vi "py.create.Pitch.vi"(8 "error in (no error)":errorcluster, 11 "Parameters":variant) -> (0 "error out":errorcluster, 3 "bytes":u8[](array[numeric]) format="%.0x")   [LabVIEW 2020]
uses:
  AddOrder/AddOrderLong.Parameters.ctl
  Time/Time.Parameters.ctl
  OrderExecuted/OrderExecuted.Parameters.ctl
  ReduceSize/ReduceSizeLong.Parameters.ctl
  ReduceSize/ReduceSizeShort.Parameters.ctl
  ModifyOrder/ModifyOrderLong.Parameters.ctl
  ModifyOrder/ModifyOrderShort.Parameters.ctl
  DeleteOrder/DeleteOrder.Parameters.ctl
  Trade/TradeLong.Parameters.ctl
  Trade/TradeShort.Parameters.ctl
  Trade/TradeExpanded.Parameters.ctl
  AddOrder/AddOrderShort.Parameters.ctl
  AddOrder/AddOrderExpanded.Parameters.ctl
  OrderExecuted/OrderExecutedAtPriceSize.Parameters.ctl
  <vilib>/Utility/Data Type/NI_Data Type.lvlib
  AddOrder/AddOrderLong.lvclass
  Time/Time.lvclass
  OrderExecuted/OrderExecuted.lvclass
  ReduceSize/ReduceSizeLong.lvclass
  ReduceSize/ReduceSizeShort.lvclass
  ModifyOrder/ModifyOrderLong.lvclass
  ModifyOrder/ModifyOrderShort.lvclass
  DeleteOrder/DeleteOrder.lvclass
  Trade/TradeLong.lvclass
  Trade/TradeShort.lvclass
  Trade/TradeExpanded.lvclass
  AddOrder/AddOrderShort.lvclass
  AddOrder/AddOrderExpanded.lvclass
  OrderExecuted/OrderExecutedAtPriceSize.lvclass
panel:
  out "Application Directory":path
  out "name":string
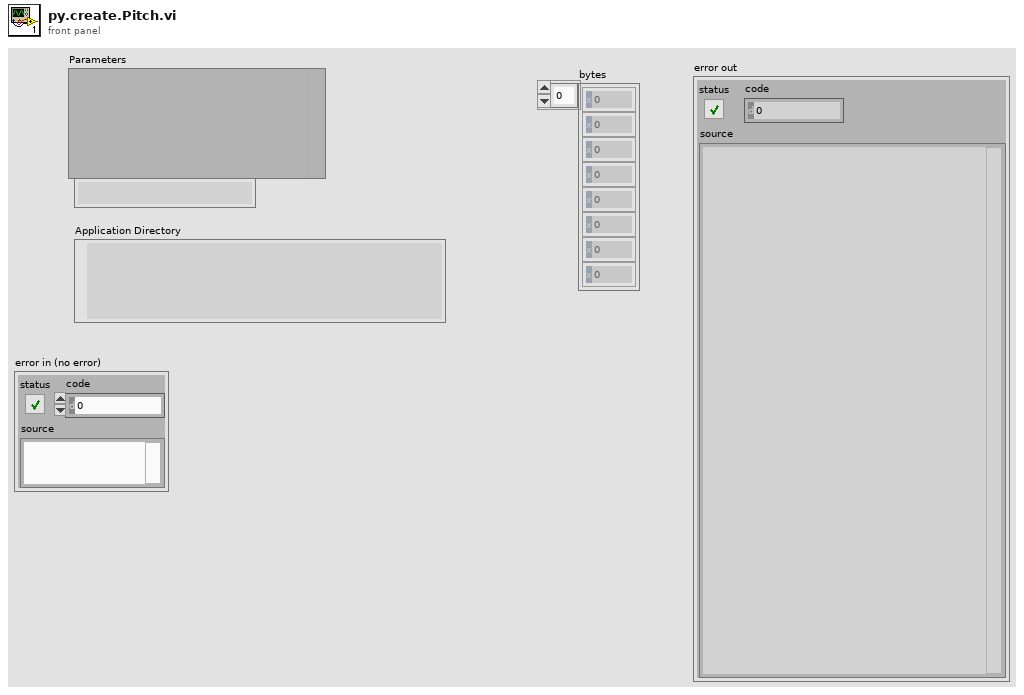
[diagram p1: front panel]
types:
  T1 = typedef "AddOrderLong.lvclass/AddOrderLong.Parameters.ctl" = cluster{"Time Offset":u32, "Order Id":string, "Quantity":u32, "Symbol":string, "Side Indicator":string, "Price":dbl}
  T2 = typedef "Time.lvclass/Time.Parameters.ctl" = cluster{"Time":u32}
  T3 = typedef "OrderExecuted.lvclass/OrderExecuted.Parameters.ctl" = cluster{"Time Offset":u32, "Order Id":string, "Executed Quantity":u32, "Execution Id":string}
  T4 = typedef "ReduceSizeLong.lvclass/ReduceSizeLong.Parameters.ctl" = cluster{"Time Offset":u32, "Order Id":string, "Canceled Quantity":u32}
  T5 = typedef "ReduceSizeShort.lvclass/ReduceSizeShort.Parameters.ctl" = cluster{"Time Offset":u32, "Order Id":string, "Canceled Quantity":u16}
  T6 = typedef "ModifyOrderLong.lvclass/ModifyOrderLong.Parameters.ctl" = cluster{"Time Offset":u32, "Order Id":string, "Quantity":u32, "Price":dbl, "Modify Flags":u8}
  T7 = typedef "ModifyOrderShort.lvclass/ModifyOrderShort.Parameters.ctl" = cluster{"Time Offset":u32, "Order Id":string, "Quantity":u32, "Price":u16, "Modify Flags":u8}
  T8 = typedef "DeleteOrder.lvclass/DeleteOrder.Parameters.ctl" = cluster{"Time Offset":u32, "Order Id":string}
  T9 = typedef "TradeLong.lvclass/TradeLong.Parameters.ctl" = cluster{"Time Offset":u32, "Order Id":string, "Execution Id":string, "Quantity":u32, "Price":dbl, "Side Indicator":string, "Symbol":string}
  T10 = typedef "TradeShort.lvclass/TradeShort.Parameters.ctl" = cluster{"Time Offset":u32, "Order Id":string, "Execution Id":string, "Quantity":u32, "Price":dbl, "Side Indicator":string, "Symbol":string}
  T11 = typedef "TradeExpanded.lvclass/TradeExpanded.Parameters.ctl" = cluster{"Time Offset":u32, "Order Id":string, "Side Indicator":string, "Quantity":u32, "Symbol":string, "Price":dbl, "Execution Id":string}
  T12 = typedef "AddOrderShort.lvclass/AddOrderShort.Parameters.ctl" = cluster{"Time Offset":u32, "Order Id":string, "Quantity":u32, "Symbol":string, "Side Indicator":string, "Price":dbl}
  T13 = typedef "AddOrderExpanded.lvclass/AddOrderExpanded.Parameters.ctl" = cluster{"Time Offset":u32, "Order Id":string, "Quantity":u32, "Symbol":string, "Side Indicator":string, "Price":dbl, "Participant Id":string, "Customer Indicator":string}
  T14 = typedef "OrderExecutedAtPriceSize.lvclass/OrderExecutedAtPriceSize.Parameters.ctl" = cluster{"Time Offset":u32, "Order Id":string, "Executed Quantity":u32, "Execution Id":string, "Remaining Quantity":u32, "Price":dbl}
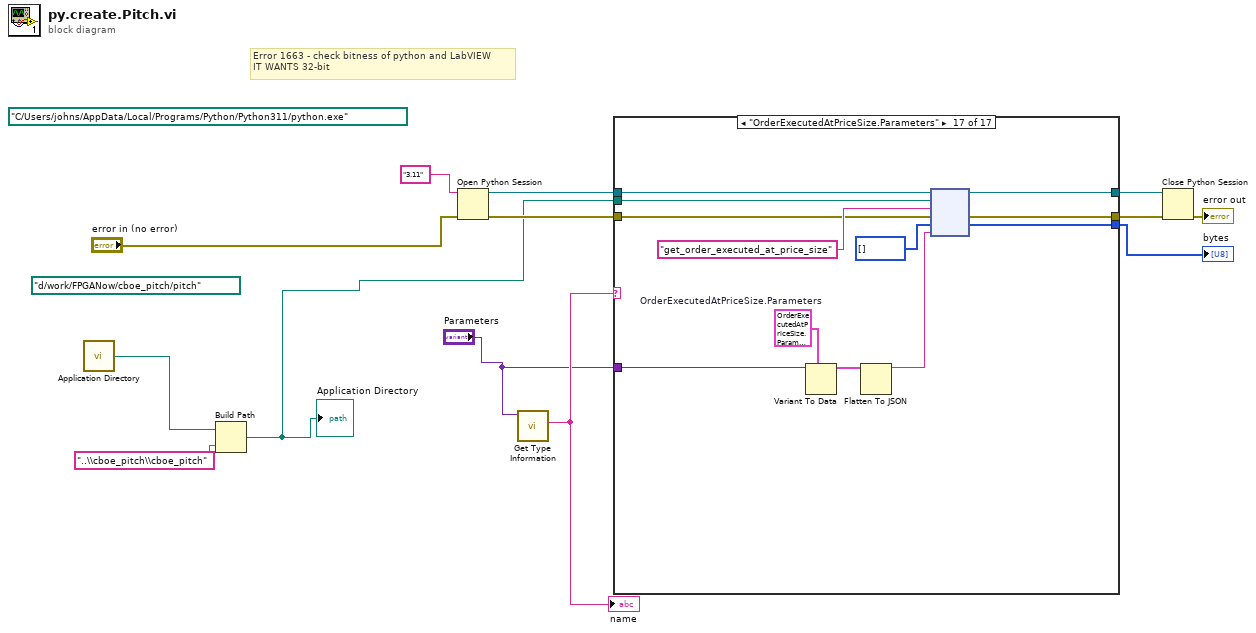
[diagram p0: block diagram]
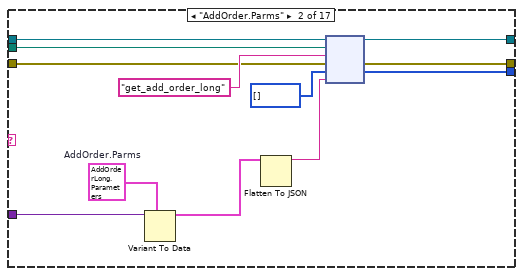
[diagram p3: hidden frame]
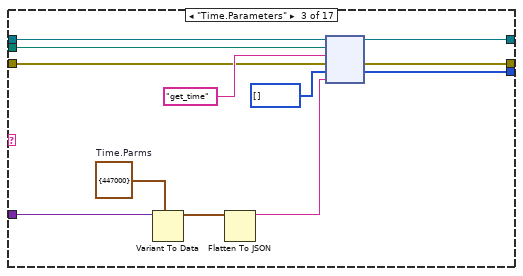
[diagram p4: hidden frame]
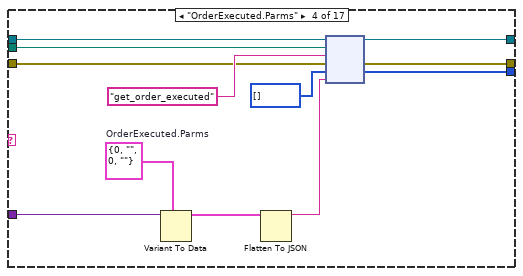
[diagram p5: hidden frame]
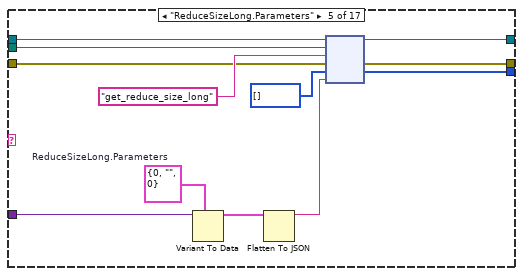
[diagram p6: hidden frame]
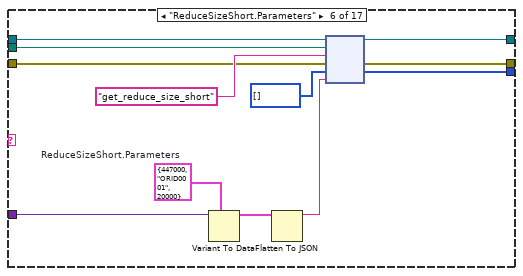
[diagram p7: hidden frame]
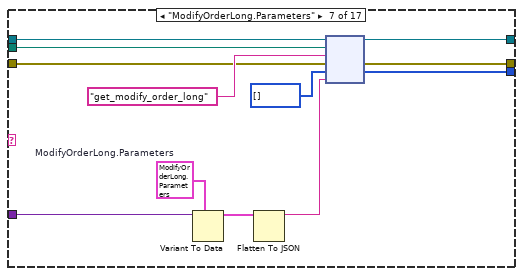
[diagram p8: hidden frame]
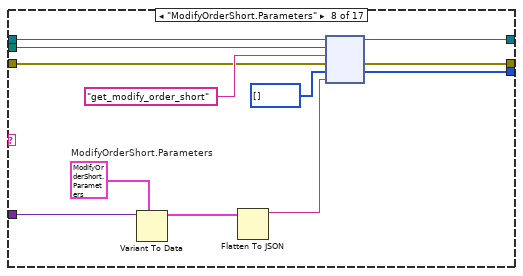
[diagram p9: hidden frame]
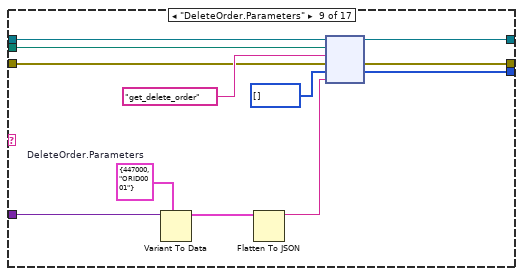
[diagram p10: hidden frame]
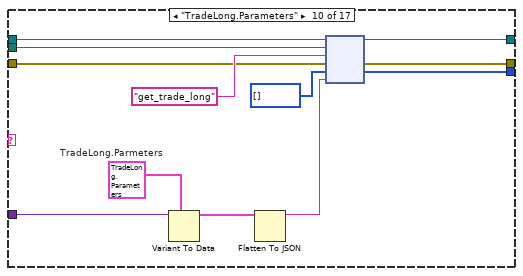
[diagram p11: hidden frame]
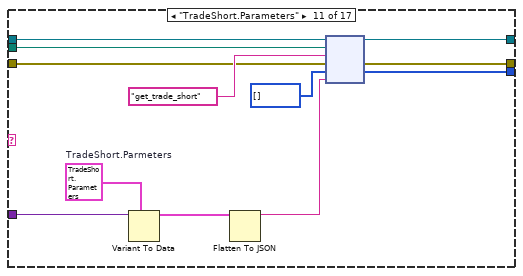
[diagram p12: hidden frame]
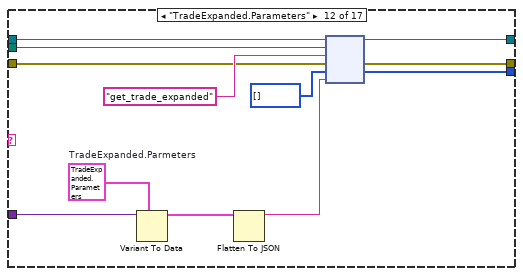
[diagram p13: hidden frame]
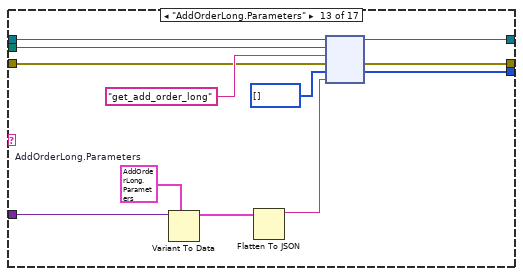
[diagram p14: hidden frame]
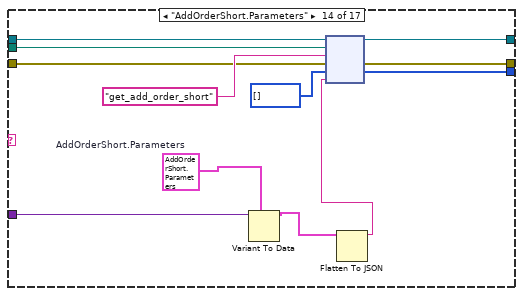
[diagram p15: hidden frame]
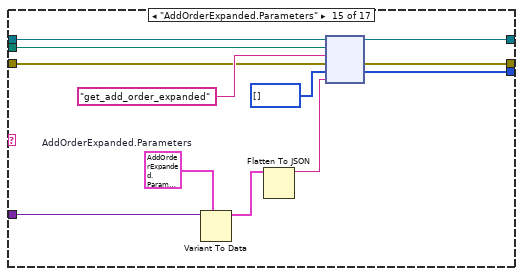
[diagram p16: hidden frame]
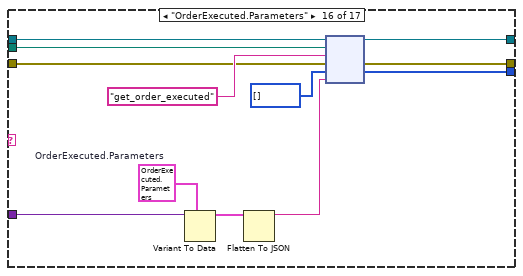
[diagram p17: hidden frame]
diagram:
  (unwired) path "C:/Users/johns/AppData/Local/Programs/Python/Python311/python.exe" ("Python path")
  (unwired) path "d:/work/FPGANow/cboe_pitch/pitch" ("module path")
  # "Error 1663 - check bitness of python and LabVIEW\nIT WANTS 32-bit"
  n1 = call <vilib>:"Application Directory.vi"() -> ("Application Directory"=w6:path)
  n2 = Build Path(base path=w6, name or relative path="..\\cboe_pitch\\cboe_pitch") -> (appended path=w4:path)
  "Application Directory" <- w4
  n3 = Open Python Session(python version="3.11" ("Python version"), 3:"error in (no error)") -> (session out=w3:refnum<k35>, error out=w10:errorcluster)  [unwired: 1 in]
  n4 = call <vilib>:"Get Type Information.vi"("variant"="Parameters") -> ("name"=w2:string)  [unwired: 6 in, 4 out]
  "name" <- w2
  n5 = case shown="\"OrderExecutedAtPriceSize.Parameters\"" w2 {
    tunnel: w3 -> [w15 w27 w39 w51 w63 w75 w87 w99 w111 w123 w135 w147 w159 w171 w183 w195 w207]
    tunnel: [w15 w26 w38 w50 w62 w74 w86 w98 w110 w122 w134 w146 w158 w170 w182 w194 w206] -> w13
    tunnel: w4 -> [_ w25 w37 w49 w61 w73 w85 w97 w109 w121 w133 w145 w157 w169 w181 w193 w205]
    tunnel: [w14 w24 w36 w48 w60 w72 w84 w96 w108 w120 w132 w144 w156 w168 w180 w192 w204] -> w11
    tunnel: w10 -> [w14 w22 w34 w46 w58 w70 w82 w94 w106 w118 w130 w142 w154 w166 w178 w190 w202]
    tunnel: [_ w21 w33 w45 w57 w69 w81 w93 w105 w117 w129 w141 w153 w165 w177 w189 w201] -> w9
    tunnel: "Parameters" -> [_ w19 w31 w43 w55 w67 w79 w91 w103 w115 w127 w139 w151 w163 w174 w187 w199]
    frame "False", Default {
    }
    frame "AddOrder.Parms" {
      w18 = T1 {"Time Offset"=447000, "Order Id"="ORID0001", "Quantity"=20000, "Symbol"="AAPL", "Side Indicator"="B", "Price"=0.905}  # AddOrder.Parms
      n6 = Variant To Data(type=w18, Variant=w19) -> (data=w17:T1)  [unwired: 1 in, 1 out]
      n7 = Flatten To JSON(anything=w17) -> (JSON string=w16:string)  [unwired: 2 in, 1 out]
      n8 = node(w27, w25, "get_add_order_long" ("function name"), w22, u8[] [], w16) -> (w26:refnum<k35>, w24:errorcluster, w21:u8[])  [unwired: 1 in, 2 out]
    }
    frame "Time.Parameters" {
      w30 = T2 {"Time"=447000}  # Time.Parms
      n9 = Variant To Data(type=w30, Variant=w31) -> (data=w29:T2)  [unwired: 1 in, 1 out]
      n10 = Flatten To JSON(anything=w29) -> (JSON string=w28:string)  [unwired: 2 in, 1 out]
      n11 = node(w39, w37, "get_time" ("function name"), w34, u8[] [], w28) -> (w38:refnum<k35>, w36:errorcluster, w33:u8[])  [unwired: 1 in, 2 out]
    }
    frame "OrderExecuted.Parms" {
      w42 = T3 {"Time Offset"=0, "Order Id"="", "Executed Quantity"=0, "Execution Id"=""}  # OrderExecuted.Parms
      n12 = Variant To Data(type=w42, Variant=w43) -> (data=w41:T3)  [unwired: 1 in, 1 out]
      n13 = Flatten To JSON(anything=w41) -> (JSON string=w40:string)  [unwired: 2 in, 1 out]
      n14 = node(w51, w49, "get_order_executed" ("function name"), w46, u8[] [], w40) -> (w50:refnum<k35>, w48:errorcluster, w45:u8[])  [unwired: 1 in, 2 out]
    }
    frame "ReduceSizeLong.Parameters" {
      w54 = T4 {"Time Offset"=0, "Order Id"="", "Canceled Quantity"=0}  # ReduceSizeLong.Parameters
      n15 = Variant To Data(type=w54, Variant=w55) -> (data=w53:T4)  [unwired: 1 in, 1 out]
      n16 = Flatten To JSON(anything=w53) -> (JSON string=w52:string)  [unwired: 2 in, 1 out]
      n17 = node(w63, w61, "get_reduce_size_long" ("function name"), w58, u8[] [], w52) -> (w62:refnum<k35>, w60:errorcluster, w57:u8[])  [unwired: 1 in, 2 out]
    }
    frame "ReduceSizeShort.Parameters" {
      w66 = T5 {"Time Offset"=447000, "Order Id"="ORID0001", "Canceled Quantity"=20000}  # ReduceSizeShort.Parameters
      n18 = Variant To Data(type=w66, Variant=w67) -> (data=w65:T5)  [unwired: 1 in, 1 out]
      n19 = Flatten To JSON(anything=w65) -> (JSON string=w64:string)  [unwired: 2 in, 1 out]
      n20 = node(w75, w73, "get_reduce_size_short" ("function name"), w70, u8[] [], w64) -> (w74:refnum<k35>, w72:errorcluster, w69:u8[])  [unwired: 1 in, 2 out]
    }
    frame "ModifyOrderLong.Parameters" {
      w78 = T6 {"Time Offset"=447000, "Order Id"="ORID0001", "Quantity"=20000, "Price"=0.905, "Modify Flags"=1}  # ModifyOrderLong.Parameters
      n21 = Variant To Data(type=w78, Variant=w79) -> (data=w77:T6)  [unwired: 1 in, 1 out]
      n22 = Flatten To JSON(anything=w77) -> (JSON string=w76:string)  [unwired: 2 in, 1 out]
      n23 = node(w87, w85, "get_modify_order_long" ("function name"), w82, u8[] [], w76) -> (w86:refnum<k35>, w84:errorcluster, w81:u8[])  [unwired: 1 in, 2 out]
    }
    frame "ModifyOrderShort.Parameters" {
      w90 = T7 {"Time Offset"=447000, "Order Id"="ORID0001", "Quantity"=20000, "Price"=1, "Modify Flags"=1}  # ModifyOrderShort.Parameters
      n24 = Variant To Data(type=w90, Variant=w91) -> (data=w89:T7)  [unwired: 1 in, 1 out]
      n25 = Flatten To JSON(anything=w89) -> (JSON string=w88:string)  [unwired: 2 in, 1 out]
      n26 = node(w99, w97, "get_modify_order_short" ("function name"), w94, u8[] [], w88) -> (w98:refnum<k35>, w96:errorcluster, w93:u8[])  [unwired: 1 in, 2 out]
    }
    frame "DeleteOrder.Parameters" {
      w102 = T8 {"Time Offset"=447000, "Order Id"="ORID0001"}  # DeleteOrder.Parameters
      n27 = Variant To Data(type=w102, Variant=w103) -> (data=w101:T8)  [unwired: 1 in, 1 out]
      n28 = Flatten To JSON(anything=w101) -> (JSON string=w100:string)  [unwired: 2 in, 1 out]
      n29 = node(w111, w109, "get_delete_order" ("function name"), w106, u8[] [], w100) -> (w110:refnum<k35>, w108:errorcluster, w105:u8[])  [unwired: 1 in, 2 out]
    }
    frame "TradeLong.Parameters" {
      w114 = T9 {"Time Offset"=447000, "Order Id"="ORID0001", "Execution Id"="EXE_ID_1", "Quantity"=20000, "Price"=0.905, "Side Indicator"="B", "Symbol"="AAPL"}  # TradeLong.Parmeters
      n30 = Variant To Data(type=w114, Variant=w115) -> (data=w113:T9)  [unwired: 1 in, 1 out]
      n31 = Flatten To JSON(anything=w113) -> (JSON string=w112:string)  [unwired: 2 in, 1 out]
      n32 = node(w123, w121, "get_trade_long" ("function name"), w118, u8[] [], w112) -> (w122:refnum<k35>, w120:errorcluster, w117:u8[])  [unwired: 1 in, 2 out]
    }
    frame "TradeShort.Parameters" {
      w126 = T10 {"Time Offset"=447000, "Order Id"="ORID0001", "Execution Id"="EXE_ID_1", "Quantity"=20000, "Price"=0.905, "Side Indicator"="B", "Symbol"="AAPL"}  # TradeShort.Parmeters
      n33 = Variant To Data(type=w126, Variant=w127) -> (data=w125:T10)  [unwired: 1 in, 1 out]
      n34 = Flatten To JSON(anything=w125) -> (JSON string=w124:string)  [unwired: 2 in, 1 out]
      n35 = node(w135, w133, "get_trade_short" ("function name"), w130, u8[] [], w124) -> (w134:refnum<k35>, w132:errorcluster, w129:u8[])  [unwired: 1 in, 2 out]
    }
    frame "TradeExpanded.Parameters" {
      w138 = T11 {"Time Offset"=447000, "Order Id"="ORID0001", "Side Indicator"="B", "Quantity"=20000, "Symbol"="AAPL", "Price"=0.905, "Execution Id"="EXE_ID_1"}  # TradeExpanded.Parmeters
      n36 = Variant To Data(type=w138, Variant=w139) -> (data=w137:T11)  [unwired: 1 in, 1 out]
      n37 = Flatten To JSON(anything=w137) -> (JSON string=w136:string)  [unwired: 2 in, 1 out]
      n38 = node(w147, w145, "get_trade_expanded" ("function name"), w142, u8[] [], w136) -> (w146:refnum<k35>, w144:errorcluster, w141:u8[])  [unwired: 1 in, 2 out]
    }
    frame "AddOrderLong.Parameters" {
      w150 = T1 {"Time Offset"=447000, "Order Id"="ORID0001", "Quantity"=20000, "Symbol"="AAPL", "Side Indicator"="B", "Price"=0.905}  # AddOrderLong.Parameters
      n39 = Variant To Data(type=w150, Variant=w151) -> (data=w149:T1)  [unwired: 1 in, 1 out]
      n40 = Flatten To JSON(anything=w149) -> (JSON string=w148:string)  [unwired: 2 in, 1 out]
      n41 = node(w159, w157, "get_add_order_long" ("function name"), w154, u8[] [], w148) -> (w158:refnum<k35>, w156:errorcluster, w153:u8[])  [unwired: 1 in, 2 out]
    }
    frame "AddOrderShort.Parameters" {
      w162 = T12 {"Time Offset"=447000, "Order Id"="ORID0001", "Quantity"=20000, "Symbol"="AAPL", "Side Indicator"="B", "Price"=0.905}  # AddOrderShort.Parameters
      n42 = Variant To Data(type=w162, Variant=w163) -> (data=w161:T12)  [unwired: 1 in, 1 out]
      n43 = Flatten To JSON(anything=w161) -> (JSON string=w160:string)  [unwired: 2 in, 1 out]
      n44 = node(w171, w169, "get_add_order_short" ("function name"), w166, u8[] [], w160) -> (w170:refnum<k35>, w168:errorcluster, w165:u8[])  [unwired: 1 in, 2 out]
    }
    frame "AddOrderExpanded.Parameters" {
      w175 = T13 {"Time Offset"=447000, "Order Id"="ORID0001", "Quantity"=20000, "Symbol"="AAPL", "Side Indicator"="B", "Price"=0.905, "Participant Id"="B", "Customer Indicator"="B"}  # AddOrderExpanded.Parameters
      n45 = Variant To Data(type=w175, Variant=w174) -> (data=w173:T13)  [unwired: 1 in, 1 out]
      n46 = Flatten To JSON(anything=w173) -> (JSON string=w172:string)  [unwired: 2 in, 1 out]
      n47 = node(w183, w181, "get_add_order_expanded" ("function name"), w178, u8[] [], w172) -> (w182:refnum<k35>, w180:errorcluster, w177:u8[])  [unwired: 1 in, 2 out]
    }
    frame "OrderExecuted.Parameters" {
      w186 = T3 {"Time Offset"=447000, "Order Id"="ORID0001", "Executed Quantity"=20000, "Execution Id"="AAPL"}  # OrderExecuted.Parameters
      n48 = Variant To Data(type=w186, Variant=w187) -> (data=w185:T3)  [unwired: 1 in, 1 out]
      n49 = Flatten To JSON(anything=w185) -> (JSON string=w184:string)  [unwired: 2 in, 1 out]
      n50 = node(w195, w193, "get_order_executed" ("function name"), w190, u8[] [], w184) -> (w194:refnum<k35>, w192:errorcluster, w189:u8[])  [unwired: 1 in, 2 out]
    }
    frame "OrderExecutedAtPriceSize.Parameters" {
      w198 = T14 {"Time Offset"=447000, "Order Id"="ORID0001", "Executed Quantity"=20000, "Execution Id"="AAPL", "Remaining Quantity"=20000, "Price"=0.905}  # OrderExecutedAtPriceSize.Parameters
      n51 = Variant To Data(type=w198, Variant=w199) -> (data=w197:T14)  [unwired: 1 in, 1 out]
      n52 = Flatten To JSON(anything=w197) -> (JSON string=w196:string)  [unwired: 2 in, 1 out]
      n53 = node(w207, w205, "get_order_executed_at_price_size" ("function name"), w202, u8[] [], w196) -> (w206:refnum<k35>, w204:errorcluster, w201:u8[])  [unwired: 1 in, 2 out]
    }
  }
  "bytes" <- w9
  n54 = Close Python Session(session in=w13, error in=w11) -> (11:→"error out":errorcluster)
